vi "IMAQ FPGA Wait for Image Transfer Complete.vi"   [LabVIEW 2020, in "NI_VDM_FPGA_Basics.lvlib"]
doc: "Waits for the transfer of image data from the host processor to the target FPGA via a DMA FIFO to complete or for the specified timeout to expire before returning. The transfer is deemed complete when the host-side buffer of the DMA FIFO is empty and the DMA FIFO on the FPGA is empty as well. To ensure that none of the image data will be lost, call this VI after the last call to the IMAQ FPGA Image Transfer to Target VI and prior to calling the Close FPGA VI Reference function on the DMA FIFO Reference."
uses:
  <vilib>/visionFPGA/NI_VDM_FPGA_Basics.lvlib
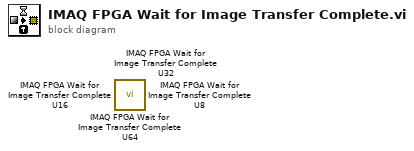
[diagram p0: block diagram]
diagram:
  n1 = call <vilib>:"IMAQ FPGA Wait for Image Transfer Complete U64.vi"() -> ()  [unwired: 10 in, 2 out]
  n2 = call <vilib>:"IMAQ FPGA Wait for Image Transfer Complete U32.vi"() -> ()  [unwired: 10 in, 2 out]
  n3 = call <vilib>:"IMAQ FPGA Wait for Image Transfer Complete U16.vi"() -> ()  [unwired: 10 in, 2 out]
  n4 = call <vilib>:"IMAQ FPGA Wait for Image Transfer Complete U8.vi"() -> ()  [unwired: 10 in, 2 out]
